vi "Update String Values.vi"(8 "error in (no error)":errorcluster, 10 "Type":u16, 11 "Rigol DG822 Pulse in":refnum<class "Rigol DG822 Pulse.lvclass">) -> (0 "error out":errorcluster, 3 "Rigol DG822 Pulse out":refnum<class "Rigol DG822 Pulse.lvclass">)   [LabVIEW 2021, in "Rigol DG822 UI.lvlib" / "Rigol DG822 Pulse.lvlib" / "Rigol DG822 Pulse.lvclass"]
uses:
  Rigol DG822 Pulse.lvclass
  Rigol DG822 UI/lib/controls.llb/WaveformExtCall.ctl
  Rigol DG822 Pulse.lvclass/Rigol DG822 Pulse.ctl
  General/Files/lvlibp/Actors.lvlibp/Actors/Actors/Actors.lvclass
  D:/LabVIEW/General/Files/lvlibp/Actors.lvlibp/Actors/Actors/Actors.lvclass
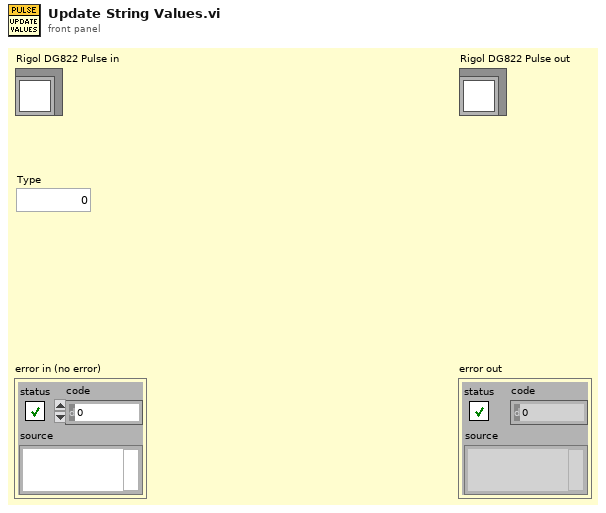
[diagram p1: front panel]
types:
  T1 = cluster{"Freq-Period":string, "Freq-Period 2":string, "Freq-Period 3":string, "Freq-Period 4":string, "Freq-Period 5":string, "Freq-Period 6":string, "Freq-Period 7":string}
  T2 = typedef "WaveformExtCall.ctl" = enum16{"Freq", "Period", "Ampl", "HighL", "Offset", "LowL", "Phase", "Duty", "Width", "RisEdge", "FallEdge", "Home", "InitData"}
  T3 = cluster{"Control Label":string, "Control Label 2":string, "Control Label 3":string, "Control Label 4":string}
  T4 = enum32{"No Selection", "MHz", "kHz", "Hz", "mHz", "uHz"}
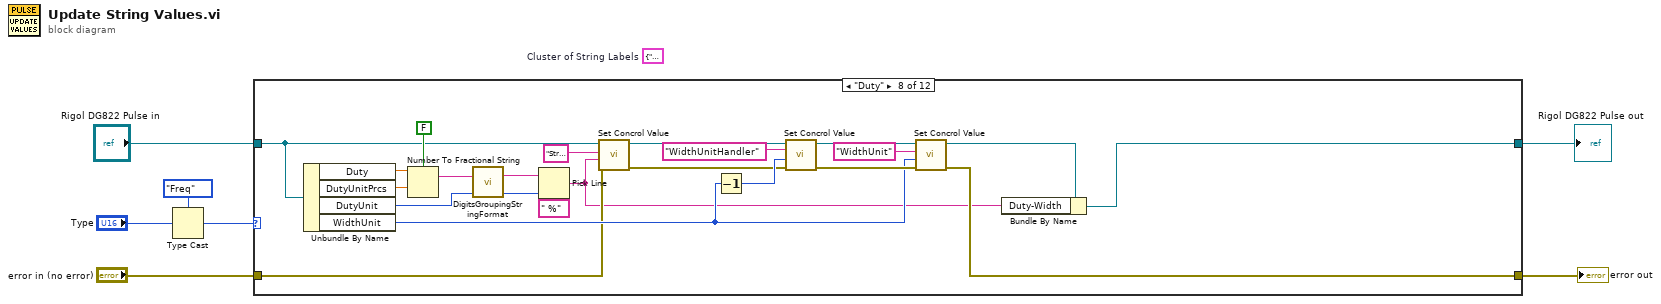
[diagram p0: block diagram]
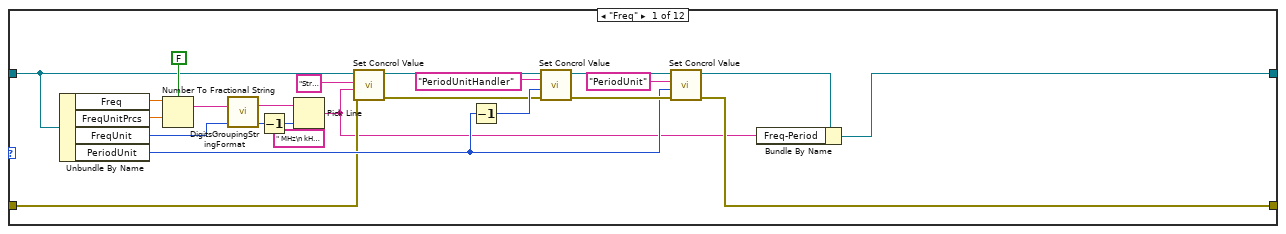
[diagram p2: hidden frame]
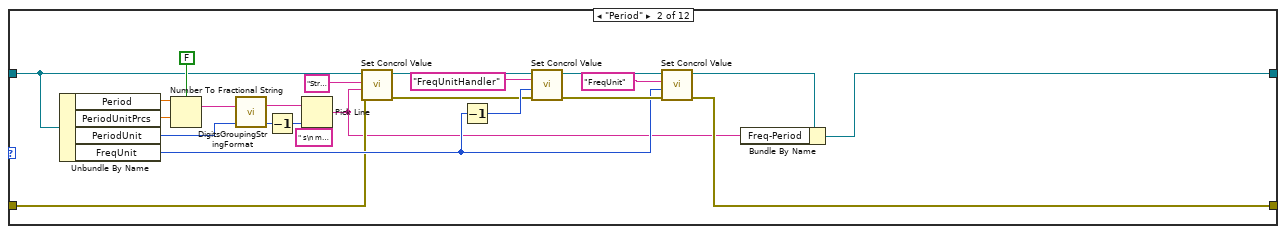
[diagram p3: hidden frame]
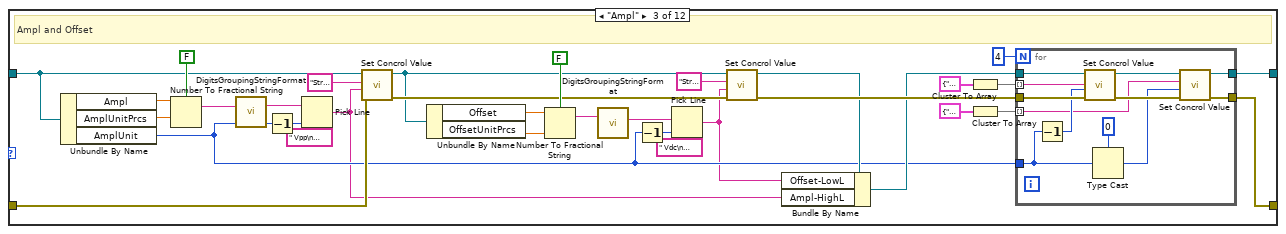
[diagram p4: hidden frame]
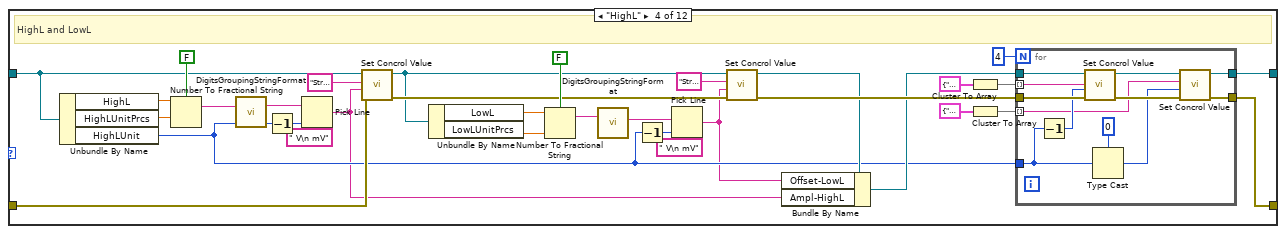
[diagram p5: hidden frame]
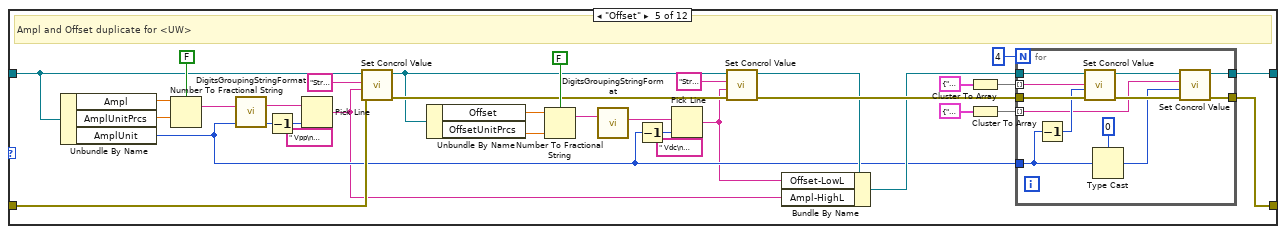
[diagram p6: hidden frame]
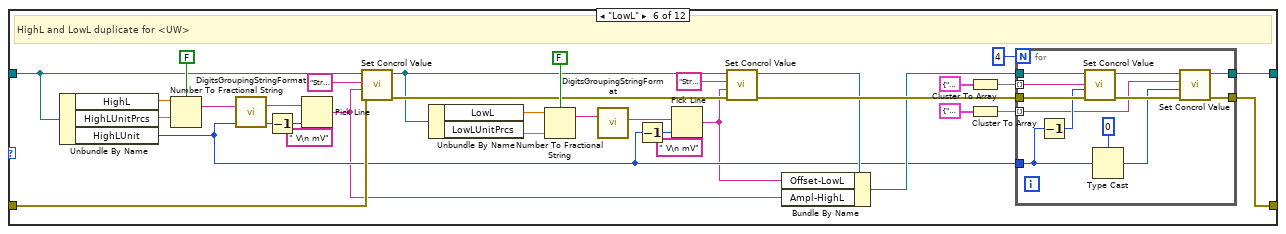
[diagram p7: hidden frame]
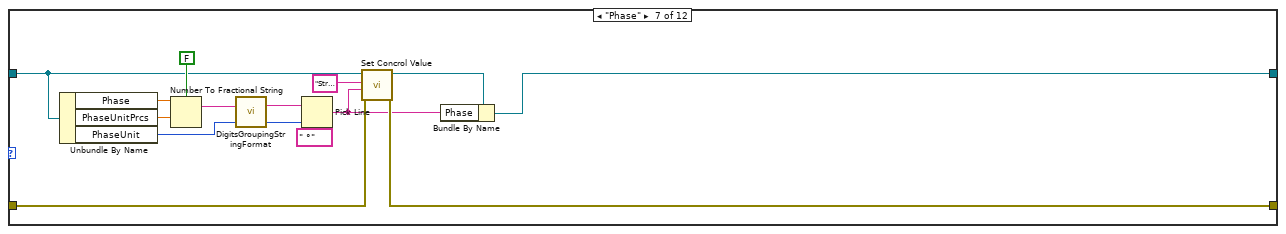
[diagram p8: hidden frame]
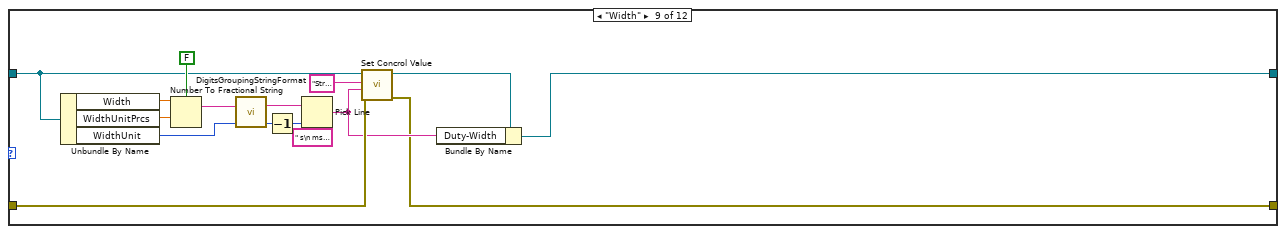
[diagram p9: hidden frame]
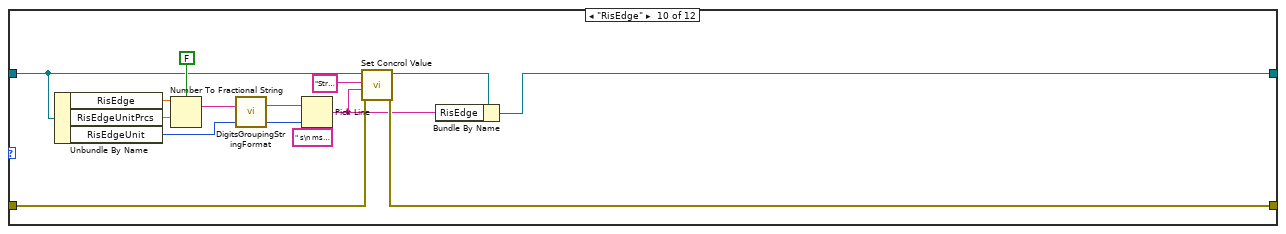
[diagram p10: hidden frame]
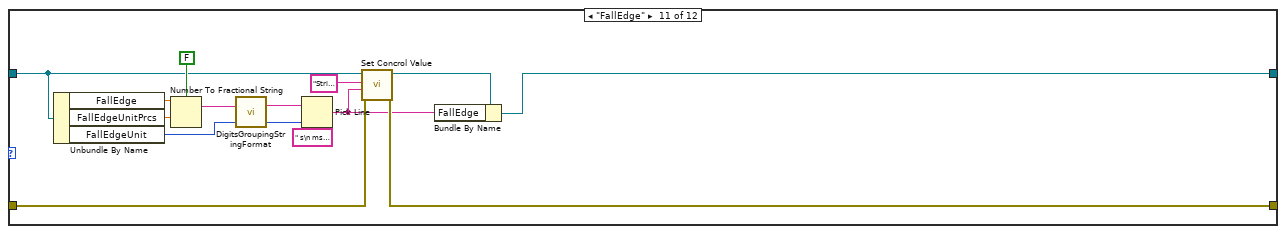
[diagram p11: hidden frame]
diagram:
  (unwired) T1 {"Freq-Period"="String Indcs.Freq-Period", "Freq-Period 2"="String Indcs.Ampl-HighL", "Freq-Period 3"="String Indcs.Offset-LowL", "Freq-Period 4"="String Indcs.Phase", "Freq-Period 5"="String Indcs 2.Duty-Width", "Freq-Period 6"="String Indcs 2.RisEdge", "Freq-Period 7"="String Indcs 2.Falldge"}  # Cluster of String Labels
  n1 = Type Cast(type=WaveformExtCall."Freq" ("SineExtCall"), x="Type") -> (*(type *) &x=w4:T2)
  n2 = case shown="\"Duty\"" w4 {
    tunnel: "error in (no error)" -> [w16 w39 w64 w111 w154 w201 w239 w255 w277 w291 w305 w313]
    tunnel: [w10 w32 w70 w116 w160 w206 w235 w251 w273 w287 w301 w314] -> w3
    tunnel: [w14 w37 w75 w121 w165 w211 w237 w253 w270 w289 w303 w313] -> w1
    tunnel: "Rigol DG822 Pulse in" -> [w8 w43 w77 w123 w167 w213 w242 w249 w280 w294 w308 w314]
    frame "Freq" {
      n3 = Unbundle By Name(w8) -> ("Freq"=w17:dbl, "FreqUnitPrcs"=w18:dbl, "FreqUnit"=w13:T4, "PeriodUnit"=w19:enum32{"No Selection", "s", "ms", "us", "ns"})
      n4 = Number To Fractional String(use system decimal point (T)=FALSE, number=w17, precision (6)=w18) -> (F-format string=w30:string)  [unwired: 1 in]
      n5 = call "DigitsGroupingStringFormat.vi"("Input string"=w30) -> ("Digit grouped string"=w29:string)  [unwired: 8 in, 2 out]
      n6 = Decrement(x=w13) -> (x-1=w12:T4)
      n7 = Pick Line(string ("")=w29, multi-line string=" MHz\n kHz\n Hz\n mHz\n uHz", line index=w12) -> (output string=w9:string)
      n8 = call "Set Concrol Value.vi"("error in (no error)"=w16, "Value"=w9, "Control Label"="String Indcs.Freq-Period", "Actors in"=w8) -> ("error out"=w15:errorcluster, "Actors out"=w28:refnum<class "Rigol DG822 Pulse.lvclass">)  [unwired: 6 in]
      n9 = Decrement(x=w19) -> (x-1=w26:enum32{"No Selection", "s", "ms", "us", "ns"})
      n10 = call "Set Concrol Value.vi"("error in (no error)"=w15, "Value"=w26, "Control Label"="PeriodUnitHandler", "Actors in"=w28) -> ("error out"=w25:errorcluster, "Actors out"=w27:refnum<class "Rigol DG822 Pulse.lvclass">)  [unwired: 6 in]
      n11 = call "Set Concrol Value.vi"("error in (no error)"=w25, "Value"=w19, "Control Label"="PeriodUnit", "Actors in"=w27) -> ("error out"=w14:errorcluster, "Actors out"=w11:refnum<class "Rigol DG822 Pulse.lvclass">)  [unwired: 6 in]
      n12 = Bundle By Name(cluster=w11, "Freq-Period"=w9) -> (w10:refnum<class "Rigol DG822 Pulse.lvclass">)
    }
    frame "Period" {
      n13 = Unbundle By Name(w43) -> ("Period"=w40:dbl, "PeriodUnitPrcs"=w41:dbl, "PeriodUnit"=w34:enum32{"No Selection", "s", "ms", "us", "ns"}, "FreqUnit"=w42:T4)
      n14 = Number To Fractional String(use system decimal point (T)=FALSE, number=w40, precision (6)=w41) -> (F-format string=w53:string)  [unwired: 1 in]
      n15 = call "DigitsGroupingStringFormat.vi"("Input string"=w53) -> ("Digit grouped string"=w52:string)  [unwired: 8 in, 2 out]
      n16 = Decrement(x=w34) -> (x-1=w35:enum32{"No Selection", "s", "ms", "us", "ns"})
      n17 = Pick Line(string ("")=w52, multi-line string=" s\n ms\n us\n ns", line index=w35) -> (output string=w31:string)
      n18 = call "Set Concrol Value.vi"("error in (no error)"=w39, "Value"=w31, "Control Label"="String Indcs.Freq-Period", "Actors in"=w43) -> ("error out"=w38:errorcluster, "Actors out"=w51:refnum<class "Rigol DG822 Pulse.lvclass">)  [unwired: 6 in]
      n19 = Decrement(x=w42) -> (x-1=w49:T4)
      n20 = call "Set Concrol Value.vi"("error in (no error)"=w38, "Value"=w49, "Control Label"="FreqUnitHandler", "Actors in"=w51) -> ("error out"=w48:errorcluster, "Actors out"=w50:refnum<class "Rigol DG822 Pulse.lvclass">)  [unwired: 6 in]
      n21 = call "Set Concrol Value.vi"("error in (no error)"=w48, "Value"=w42, "Control Label"="FreqUnit", "Actors in"=w50) -> ("error out"=w37:errorcluster, "Actors out"=w33:refnum<class "Rigol DG822 Pulse.lvclass">)  [unwired: 6 in]
      n22 = Bundle By Name(cluster=w33, "Freq-Period"=w31) -> (w32:refnum<class "Rigol DG822 Pulse.lvclass">)
    }
    frame "Ampl" {
      # "Ampl and Offset"
      n23 = Unbundle By Name(w77) -> ("Ampl"=w80:dbl, "AmplUnitPrcs"=w81:dbl, "AmplUnit"=w56:enum32{"No Selection", "Vpp", "mVpp"})
      n24 = Number To Fractional String(use system decimal point (T)=FALSE, number=w80, precision (6)=w81) -> (F-format string=w84:string)  [unwired: 1 in]
      n25 = call "DigitsGroupingStringFormat.vi"("Input string"=w84) -> ("Digit grouped string"=w83:string)  [unwired: 8 in, 2 out]
      n26 = Decrement(x=w56) -> (x-1=w78:enum32{"No Selection", "Vpp", "mVpp"})
      n27 = Pick Line(string ("")=w83, multi-line string=" Vpp\n mVpp", line index=w78) -> (output string=w54:string)
      n28 = call "Set Concrol Value.vi"("error in (no error)"=w64, "Value"=w54, "Control Label"="String Indcs.Ampl-HighL", "Actors in"=w77) -> ("error out"=w60:errorcluster, "Actors out"=w59:refnum<class "Rigol DG822 Pulse.lvclass">)  [unwired: 6 in]
      n29 = Unbundle By Name(w59) -> ("Offset"=w63:dbl, "OffsetUnitPrcs"=w62:dbl)
      n30 = Number To Fractional String(use system decimal point (T)=FALSE, number=w63, precision (6)=w62) -> (F-format string=w68:string)  [unwired: 1 in]
      n31 = call "DigitsGroupingStringFormat.vi"("Input string"=w68) -> ("Digit grouped string"=w67:string)  [unwired: 8 in, 2 out]
      n32 = Decrement(x=w56) -> (x-1=w65:enum32{"No Selection", "Vpp", "mVpp"})
      n33 = Pick Line(string ("")=w67, multi-line string=" Vdc\n mVdc", line index=w65) -> (output string=w55:string)
      n34 = call "Set Concrol Value.vi"("error in (no error)"=w60, "Value"=w55, "Control Label"="String Indcs.Offset-LowL" ("Freq-Period 3"), "Actors in"=w59) -> ("error out"=w61:errorcluster, "Actors out"=w58:refnum<class "Rigol DG822 Pulse.lvclass">)  [unwired: 6 in]
      n35 = Bundle By Name(cluster=w58, "Offset-LowL"=w55, "Ampl-HighL"=w54) -> (w57:refnum<class "Rigol DG822 Pulse.lvclass">)
      n36 = Cluster To Array(cluster=T3 {"Control Label"="AmplUnitHandler", "Control Label 2"="HighLUnitHandler", "Control Label 3"="OffsetUnitHandler", "Control Label 4"="LowLUnitHandler"}) -> (array=w73:string[])
      n37 = Cluster To Array(cluster=T3 {"Control Label"="AmplUnit", "Control Label 2"="HighLUnit", "Control Label 3"="OffsetUnit", "Control Label 4"="LowLUnit"}) -> (array=w71:string[])
      n38 = for {
        N: 4 -> [_]
        tunnel: w57 -> [w97]
        tunnel: [w95] -> w70
        tunnel: [w94] -> w75
        tunnel: w61 -> [w93]
        tunnel: w73 -> [w92] mode=indexing
        tunnel: w56 -> [w87]
        tunnel: w71 -> [w90] mode=indexing
        n39 = Decrement(x=w87) -> (x-1=w91:enum32{"No Selection", "Vpp", "mVpp"})
        n40 = call "Set Concrol Value.vi"("error in (no error)"=w93, "Value"=w91, "Control Label"=w92, "Actors in"=w97) -> ("error out"=w98:errorcluster, "Actors out"=w96:refnum<class "Rigol DG822 Pulse.lvclass">)  [unwired: 6 in]
        n41 = Type Cast(type=0, x=w87) -> (*(type *) &x=w89:i32)
        n42 = call "Set Concrol Value.vi"("error in (no error)"=w98, "Value"=w89, "Control Label"=w90, "Actors in"=w96) -> ("error out"=w94:errorcluster, "Actors out"=w95:refnum<class "Rigol DG822 Pulse.lvclass">)  [unwired: 6 in]
      }
    }
    frame "HighL" {
      # "HighL and LowL"
      n43 = Unbundle By Name(w123) -> ("HighL"=w125:dbl, "HighLUnitPrcs"=w126:dbl, "HighLUnit"=w103:enum32{"No Selection", "V", "mV"})
      n44 = Number To Fractional String(use system decimal point (T)=FALSE, number=w125, precision (6)=w126) -> (F-format string=w129:string)  [unwired: 1 in]
      n45 = call "DigitsGroupingStringFormat.vi"("Input string"=w129) -> ("Digit grouped string"=w128:string)  [unwired: 8 in, 2 out]
      n46 = Decrement(x=w103) -> (x-1=w124:enum32{"No Selection", "V", "mV"})
      n47 = Pick Line(string ("")=w128, multi-line string=" V\n mV", line index=w124) -> (output string=w101:string)
      n48 = call "Set Concrol Value.vi"("error in (no error)"=w111, "Value"=w101, "Control Label"="String Indcs.Ampl-HighL", "Actors in"=w123) -> ("error out"=w107:errorcluster, "Actors out"=w106:refnum<class "Rigol DG822 Pulse.lvclass">)  [unwired: 6 in]
      n49 = Unbundle By Name(w106) -> ("LowL"=w110:dbl, "LowLUnitPrcs"=w109:dbl)
      n50 = Number To Fractional String(use system decimal point (T)=FALSE, number=w110, precision (6)=w109) -> (F-format string=w114:string)  [unwired: 1 in]
      n51 = call "DigitsGroupingStringFormat.vi"("Input string"=w114) -> ("Digit grouped string"=w113:string)  [unwired: 8 in, 2 out]
      n52 = Decrement(x=w103) -> (x-1=w112:enum32{"No Selection", "V", "mV"})
      n53 = Pick Line(string ("")=w113, multi-line string=" V\n mV", line index=w112) -> (output string=w102:string)
      n54 = call "Set Concrol Value.vi"("error in (no error)"=w107, "Value"=w102, "Control Label"="String Indcs.Offset-LowL" ("Freq-Period 3"), "Actors in"=w106) -> ("error out"=w108:errorcluster, "Actors out"=w105:refnum<class "Rigol DG822 Pulse.lvclass">)  [unwired: 6 in]
      n55 = Bundle By Name(cluster=w105, "Offset-LowL"=w102, "Ampl-HighL"=w101) -> (w104:refnum<class "Rigol DG822 Pulse.lvclass">)
      n56 = Cluster To Array(cluster=T3 {"Control Label"="AmplUnitHandler", "Control Label 2"="HighLUnitHandler", "Control Label 3"="OffsetUnitHandler", "Control Label 4"="LowLUnitHandler"}) -> (array=w119:string[])
      n57 = Cluster To Array(cluster=T3 {"Control Label"="AmplUnit", "Control Label 2"="HighLUnit", "Control Label 3"="OffsetUnit", "Control Label 4"="LowLUnit"}) -> (array=w117:string[])
      n58 = for {
        N: 4 -> [_]
        tunnel: w104 -> [w142]
        tunnel: [w140] -> w116
        tunnel: [w139] -> w121
        tunnel: w108 -> [w138]
        tunnel: w119 -> [w137] mode=indexing
        tunnel: w103 -> [w132]
        tunnel: w117 -> [w135] mode=indexing
        n59 = Decrement(x=w132) -> (x-1=w136:enum32{"No Selection", "V", "mV"})
        n60 = call "Set Concrol Value.vi"("error in (no error)"=w138, "Value"=w136, "Control Label"=w137, "Actors in"=w142) -> ("error out"=w143:errorcluster, "Actors out"=w141:refnum<class "Rigol DG822 Pulse.lvclass">)  [unwired: 6 in]
        n61 = Type Cast(type=0, x=w132) -> (*(type *) &x=w134:i32)
        n62 = call "Set Concrol Value.vi"("error in (no error)"=w143, "Value"=w134, "Control Label"=w135, "Actors in"=w141) -> ("error out"=w139:errorcluster, "Actors out"=w140:refnum<class "Rigol DG822 Pulse.lvclass">)  [unwired: 6 in]
      }
    }
    frame "Offset" {
      # "Ampl and Offset duplicate for <UW>"
      n63 = Unbundle By Name(w167) -> ("Ampl"=w170:dbl, "AmplUnitPrcs"=w171:dbl, "AmplUnit"=w146:enum32{"No Selection", "Vpp", "mVpp"})
      n64 = Number To Fractional String(use system decimal point (T)=FALSE, number=w170, precision (6)=w171) -> (F-format string=w174:string)  [unwired: 1 in]
      n65 = call "DigitsGroupingStringFormat.vi"("Input string"=w174) -> ("Digit grouped string"=w173:string)  [unwired: 8 in, 2 out]
      n66 = Decrement(x=w146) -> (x-1=w168:enum32{"No Selection", "Vpp", "mVpp"})
      n67 = Pick Line(string ("")=w173, multi-line string=" Vpp\n mVpp", line index=w168) -> (output string=w144:string)
      n68 = call "Set Concrol Value.vi"("error in (no error)"=w154, "Value"=w144, "Control Label"="String Indcs.Ampl-HighL", "Actors in"=w167) -> ("error out"=w150:errorcluster, "Actors out"=w149:refnum<class "Rigol DG822 Pulse.lvclass">)  [unwired: 6 in]
      n69 = Unbundle By Name(w149) -> ("Offset"=w153:dbl, "OffsetUnitPrcs"=w152:dbl)
      n70 = Number To Fractional String(use system decimal point (T)=FALSE, number=w153, precision (6)=w152) -> (F-format string=w158:string)  [unwired: 1 in]
      n71 = call "DigitsGroupingStringFormat.vi"("Input string"=w158) -> ("Digit grouped string"=w157:string)  [unwired: 8 in, 2 out]
      n72 = Decrement(x=w146) -> (x-1=w155:enum32{"No Selection", "Vpp", "mVpp"})
      n73 = Pick Line(string ("")=w157, multi-line string=" Vdc\n mVdc", line index=w155) -> (output string=w145:string)
      n74 = call "Set Concrol Value.vi"("error in (no error)"=w150, "Value"=w145, "Control Label"="String Indcs.Offset-LowL" ("Freq-Period 3"), "Actors in"=w149) -> ("error out"=w151:errorcluster, "Actors out"=w148:refnum<class "Rigol DG822 Pulse.lvclass">)  [unwired: 6 in]
      n75 = Bundle By Name(cluster=w148, "Offset-LowL"=w145, "Ampl-HighL"=w144) -> (w147:refnum<class "Rigol DG822 Pulse.lvclass">)
      n76 = Cluster To Array(cluster=T3 {"Control Label"="AmplUnitHandler", "Control Label 2"="HighLUnitHandler", "Control Label 3"="OffsetUnitHandler", "Control Label 4"="LowLUnitHandler"}) -> (array=w163:string[])
      n77 = Cluster To Array(cluster=T3 {"Control Label"="AmplUnit", "Control Label 2"="HighLUnit", "Control Label 3"="OffsetUnit", "Control Label 4"="LowLUnit"}) -> (array=w161:string[])
      n78 = for {
        N: 4 -> [_]
        tunnel: w147 -> [w187]
        tunnel: [w185] -> w160
        tunnel: [w184] -> w165
        tunnel: w151 -> [w183]
        tunnel: w163 -> [w182] mode=indexing
        tunnel: w146 -> [w177]
        tunnel: w161 -> [w180] mode=indexing
        n79 = Decrement(x=w177) -> (x-1=w181:enum32{"No Selection", "Vpp", "mVpp"})
        n80 = call "Set Concrol Value.vi"("error in (no error)"=w183, "Value"=w181, "Control Label"=w182, "Actors in"=w187) -> ("error out"=w188:errorcluster, "Actors out"=w186:refnum<class "Rigol DG822 Pulse.lvclass">)  [unwired: 6 in]
        n81 = Type Cast(type=0, x=w177) -> (*(type *) &x=w179:i32)
        n82 = call "Set Concrol Value.vi"("error in (no error)"=w188, "Value"=w179, "Control Label"=w180, "Actors in"=w186) -> ("error out"=w184:errorcluster, "Actors out"=w185:refnum<class "Rigol DG822 Pulse.lvclass">)  [unwired: 6 in]
      }
    }
    frame "LowL" {
      # "HighL and LowL duplicate for <UW>"
      n83 = Unbundle By Name(w213) -> ("HighL"=w215:dbl, "HighLUnitPrcs"=w216:dbl, "HighLUnit"=w193:enum32{"No Selection", "V", "mV"})
      n84 = Number To Fractional String(use system decimal point (T)=FALSE, number=w215, precision (6)=w216) -> (F-format string=w219:string)  [unwired: 1 in]
      n85 = call "DigitsGroupingStringFormat.vi"("Input string"=w219) -> ("Digit grouped string"=w218:string)  [unwired: 8 in, 2 out]
      n86 = Decrement(x=w193) -> (x-1=w214:enum32{"No Selection", "V", "mV"})
      n87 = Pick Line(string ("")=w218, multi-line string=" V\n mV", line index=w214) -> (output string=w191:string)
      n88 = call "Set Concrol Value.vi"("error in (no error)"=w201, "Value"=w191, "Control Label"="String Indcs.Ampl-HighL", "Actors in"=w213) -> ("error out"=w197:errorcluster, "Actors out"=w196:refnum<class "Rigol DG822 Pulse.lvclass">)  [unwired: 6 in]
      n89 = Unbundle By Name(w196) -> ("LowL"=w200:dbl, "LowLUnitPrcs"=w199:dbl)
      n90 = Number To Fractional String(use system decimal point (T)=FALSE, number=w200, precision (6)=w199) -> (F-format string=w204:string)  [unwired: 1 in]
      n91 = call "DigitsGroupingStringFormat.vi"("Input string"=w204) -> ("Digit grouped string"=w203:string)  [unwired: 8 in, 2 out]
      n92 = Decrement(x=w193) -> (x-1=w202:enum32{"No Selection", "V", "mV"})
      n93 = Pick Line(string ("")=w203, multi-line string=" V\n mV", line index=w202) -> (output string=w192:string)
      n94 = call "Set Concrol Value.vi"("error in (no error)"=w197, "Value"=w192, "Control Label"="String Indcs.Offset-LowL" ("Freq-Period 3"), "Actors in"=w196) -> ("error out"=w198:errorcluster, "Actors out"=w195:refnum<class "Rigol DG822 Pulse.lvclass">)  [unwired: 6 in]
      n95 = Bundle By Name(cluster=w195, "Offset-LowL"=w192, "Ampl-HighL"=w191) -> (w194:refnum<class "Rigol DG822 Pulse.lvclass">)
      n96 = Cluster To Array(cluster=T3 {"Control Label"="AmplUnitHandler", "Control Label 2"="HighLUnitHandler", "Control Label 3"="OffsetUnitHandler", "Control Label 4"="LowLUnitHandler"}) -> (array=w209:string[])
      n97 = Cluster To Array(cluster=T3 {"Control Label"="AmplUnit", "Control Label 2"="HighLUnit", "Control Label 3"="OffsetUnit", "Control Label 4"="LowLUnit"}) -> (array=w207:string[])
      n98 = for {
        N: 4 -> [_]
        tunnel: w194 -> [w232]
        tunnel: [w230] -> w206
        tunnel: [w229] -> w211
        tunnel: w198 -> [w228]
        tunnel: w209 -> [w227] mode=indexing
        tunnel: w193 -> [w222]
        tunnel: w207 -> [w225] mode=indexing
        n99 = Decrement(x=w222) -> (x-1=w226:enum32{"No Selection", "V", "mV"})
        n100 = call "Set Concrol Value.vi"("error in (no error)"=w228, "Value"=w226, "Control Label"=w227, "Actors in"=w232) -> ("error out"=w233:errorcluster, "Actors out"=w231:refnum<class "Rigol DG822 Pulse.lvclass">)  [unwired: 6 in]
        n101 = Type Cast(type=0, x=w222) -> (*(type *) &x=w224:i32)
        n102 = call "Set Concrol Value.vi"("error in (no error)"=w233, "Value"=w224, "Control Label"=w225, "Actors in"=w231) -> ("error out"=w229:errorcluster, "Actors out"=w230:refnum<class "Rigol DG822 Pulse.lvclass">)  [unwired: 6 in]
      }
    }
    frame "Phase" {
      n103 = Unbundle By Name(w242) -> ("Phase"=w240:dbl, "PhaseUnitPrcs"=w241:dbl, "PhaseUnit"=w238:enum32{"°"})
      n104 = Number To Fractional String(use system decimal point (T)=FALSE, number=w240, precision (6)=w241) -> (F-format string=w247:string)  [unwired: 1 in]
      n105 = call "DigitsGroupingStringFormat.vi"("Input string"=w247) -> ("Digit grouped string"=w246:string)  [unwired: 8 in, 2 out]
      n106 = Pick Line(string ("")=w246, multi-line string=" °", line index=w238) -> (output string=w234:string)
      n107 = call "Set Concrol Value.vi"("error in (no error)"=w239, "Value"=w234, "Control Label"="String Indcs.Phase", "Actors in"=w242) -> ("error out"=w237:errorcluster, "Actors out"=w236:refnum<class "Rigol DG822 Pulse.lvclass">)  [unwired: 6 in]
      n108 = Bundle By Name(cluster=w236, "Phase"=w234) -> (w235:refnum<class "Rigol DG822 Pulse.lvclass">)
    }
    frame "Duty" {
      n109 = Unbundle By Name(w249) -> ("Duty"=w256:dbl, "DutyUnitPrcs"=w257:dbl, "DutyUnit"=w248:enum32{"%"}, "WidthUnit"=w258:enum32{"No Selection", "s", "ms", "us", "ns"})
      n110 = Number To Fractional String(use system decimal point (T)=FALSE, number=w256, precision (6)=w257) -> (F-format string=w269:string)  [unwired: 1 in]
      n111 = call "DigitsGroupingStringFormat.vi"("Input string"=w269) -> ("Digit grouped string"=w268:string)  [unwired: 8 in, 2 out]
      n112 = Pick Line(string ("")=w268, multi-line string=" %", line index=w248) -> (output string=w250:string)
      n113 = call "Set Concrol Value.vi"("error in (no error)"=w255, "Value"=w250, "Control Label"="String Indcs 2.Duty-Width", "Actors in"=w249) -> ("error out"=w254:errorcluster, "Actors out"=w267:refnum<class "Rigol DG822 Pulse.lvclass">)  [unwired: 6 in]
      n114 = Decrement(x=w258) -> (x-1=w265:enum32{"No Selection", "s", "ms", "us", "ns"})
      n115 = call "Set Concrol Value.vi"("error in (no error)"=w254, "Value"=w265, "Control Label"="WidthUnitHandler", "Actors in"=w267) -> ("error out"=w264:errorcluster, "Actors out"=w266:refnum<class "Rigol DG822 Pulse.lvclass">)  [unwired: 6 in]
      n116 = call "Set Concrol Value.vi"("error in (no error)"=w264, "Value"=w258, "Control Label"="WidthUnit", "Actors in"=w266) -> ("error out"=w253:errorcluster, "Actors out"=w252:refnum<class "Rigol DG822 Pulse.lvclass">)  [unwired: 6 in]
      n117 = Bundle By Name(cluster=w252, "Duty-Width"=w250) -> (w251:refnum<class "Rigol DG822 Pulse.lvclass">)
    }
    frame "Width" {
      n118 = Unbundle By Name(w280) -> ("Width"=w278:dbl, "WidthUnitPrcs"=w279:dbl, "WidthUnit"=w274:enum32{"No Selection", "s", "ms", "us", "ns"})
      n119 = Number To Fractional String(use system decimal point (T)=FALSE, number=w278, precision (6)=w279) -> (F-format string=w284:string)  [unwired: 1 in]
      n120 = call "DigitsGroupingStringFormat.vi"("Input string"=w284) -> ("Digit grouped string"=w283:string)  [unwired: 8 in, 2 out]
      n121 = Decrement(x=w274) -> (x-1=w275:enum32{"No Selection", "s", "ms", "us", "ns"})
      n122 = Pick Line(string ("")=w283, multi-line string=" s\n ms\n us\n ns", line index=w275) -> (output string=w272:string)
      n123 = call "Set Concrol Value.vi"("error in (no error)"=w277, "Value"=w272, "Control Label"="String Indcs 2.Duty-Width", "Actors in"=w280) -> ("error out"=w270:errorcluster, "Actors out"=w271:refnum<class "Rigol DG822 Pulse.lvclass">)  [unwired: 6 in]
      n124 = Bundle By Name(cluster=w271, "Duty-Width"=w272) -> (w273:refnum<class "Rigol DG822 Pulse.lvclass">)
    }
    frame "RisEdge" {
      n125 = Unbundle By Name(w294) -> ("RisEdge"=w292:dbl, "RisEdgeUnitPrcs"=w293:dbl, "RisEdgeUnit"=w290:enum32{"No Selection", "s", "ms", "us", "ns"})
      n126 = Number To Fractional String(use system decimal point (T)=FALSE, number=w292, precision (6)=w293) -> (F-format string=w298:string)  [unwired: 1 in]
      n127 = call "DigitsGroupingStringFormat.vi"("Input string"=w298) -> ("Digit grouped string"=w297:string)  [unwired: 8 in, 2 out]
      n128 = Pick Line(string ("")=w297, multi-line string=" s\n ms\n us\n ns", line index=w290) -> (output string=w286:string)
      n129 = call "Set Concrol Value.vi"("error in (no error)"=w291, "Value"=w286, "Control Label"="String Indcs 2.RisEdge", "Actors in"=w294) -> ("error out"=w289:errorcluster, "Actors out"=w288:refnum<class "Rigol DG822 Pulse.lvclass">)  [unwired: 6 in]
      n130 = Bundle By Name(cluster=w288, "RisEdge"=w286) -> (w287:refnum<class "Rigol DG822 Pulse.lvclass">)
    }
    frame "FallEdge" {
      n131 = Unbundle By Name(w308) -> ("FallEdge"=w306:dbl, "FallEdgeUnitPrcs"=w307:dbl, "FallEdgeUnit"=w304:enum32{"No Selection", "s", "ms", "us", "ns"})
      n132 = Number To Fractional String(use system decimal point (T)=FALSE, number=w306, precision (6)=w307) -> (F-format string=w312:string)  [unwired: 1 in]
      n133 = call "DigitsGroupingStringFormat.vi"("Input string"=w312) -> ("Digit grouped string"=w311:string)  [unwired: 8 in, 2 out]
      n134 = Pick Line(string ("")=w311, multi-line string=" s\n ms\n us\n ns", line index=w304) -> (output string=w300:string)
      n135 = call "Set Concrol Value.vi"("error in (no error)"=w305, "Value"=w300, "Control Label"="String Indcs 2.FallEdge", "Actors in"=w308) -> ("error out"=w303:errorcluster, "Actors out"=w302:refnum<class "Rigol DG822 Pulse.lvclass">)  [unwired: 6 in]
      n136 = Bundle By Name(cluster=w302, "FallEdge"=w300) -> (w301:refnum<class "Rigol DG822 Pulse.lvclass">)
    }
    frame Default {
    }
  }
  "error out" <- w1
  "Rigol DG822 Pulse out" <- w3
